vi "Close Demo.vi"(7 "Stop Demo":refnum<user-event>, 8 "error in":errorcluster, 11 "Main Subpanel":refnum<vi>) -> (0 "error out":errorcluster)   [LabVIEW 2020]
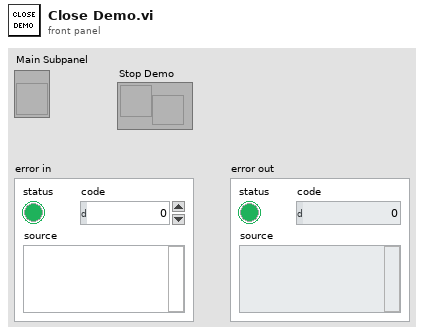
[diagram p1: front panel]
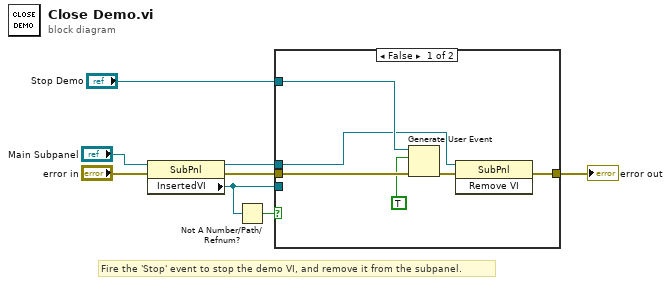
[diagram p0: block diagram]
diagram:
  # "Fire the 'Stop' event to stop the demo VI, and remove it from the subpanel."
  n1 = property class="SubPnl"(reference="Main Subpanel", error in="error in") -> (reference out=w3:refnum<vi>, error out=w7:errorcluster, "InsertedVI"=w2:refnum<vi>)
  n2 = Not A Number/Path/Refnum?(number/path/refnum=w2) -> (NaN/Path/Refnum?=w4:bool)
  n3 = case shown="False" w4 {
    tunnel: w7 -> [w13 w15]
    tunnel: w3 -> [w12 _]
    tunnel: w2 -> [_ _]
    tunnel: [w11 w15] -> w6
    tunnel: "Stop Demo" -> [w14 _]
    frame False {
      n4 = Generate User Event(user event=w14, event data cluster=TRUE ("event data"), error in=w13) -> (error out=w9:errorcluster)  [unwired: 1 in, 1 out]
      n5 = invoke class="SubPnl" method="Remove VI"(reference=w12, error in=w9) -> (error out=w11:errorcluster)  [unwired: 1 in, 2 out]
    }
    frame True {
    }
  }
  "error out" <- w6
